vi "Set simulated or real mode.vi"(8 "error in (no error)":errorcluster, 11 "Channel in":refnum<class "SPARC4_Channel.lvclass">) -> (0 "error out":errorcluster, 3 "Channel out":refnum<class "SPARC4_Channel.lvclass">)   [LabVIEW 2018, in "SPARC4_Channel.lvclass"]
doc: "Choose between the simulated or real camera class"
uses:
  SPARC4_Channel.lvclass
  C:/Users/Denis/Desktop/S4ACS/S4ACS/Channel/Channel.lvclass
  Sim_Ixon_Ultra/Sim_Ixon_Ultra.lvclass
  C:/Users/Denis/Desktop/S4ACS/S4ACS/Sim_CCD/Sim_CCD.lvclass
  Ixon_Ultra/Ixon_Ultra.lvclass
  C:/Users/Denis/Desktop/S4ACS/S4ACS/Sim_Ixon_Ultra/Sim_Ixon_Ultra.lvclass
  Channel/Channel.lvclass
  Sim_CCD/Sim_CCD.lvclass
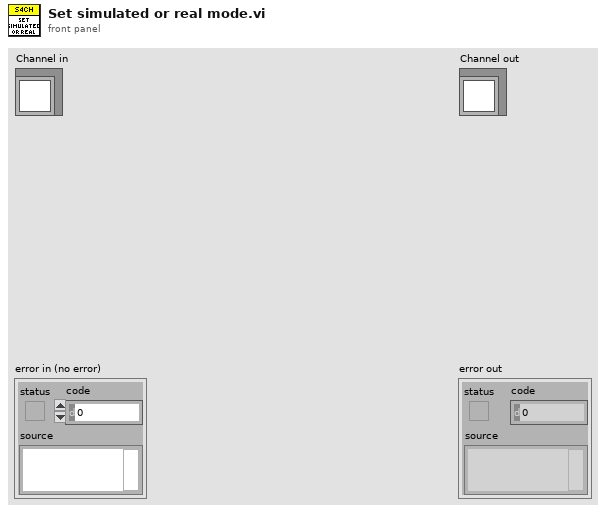
[diagram p1: front panel]
types:
  T1 = cluster{"Image path":path, "Channel":u8, "ACS mode":u16, "Log file path":path, "log level":u16}
  T2 = cluster{"State Machine.lvclass":refnum<class "State Machine.lvclass">, "RxTx.lvclass":refnum<class "RxTx.lvclass">, "Save_Header_RxTx.lvclass":refnum<class "RxTx.lvclass">, "Status SM.lvclass":refnum<class "State Machine.lvclass">, "Status RxTx.lvclass":refnum<class "RxTx.lvclass">, "servers array":refnum<class "Server.lvclass">[], "Events log file.lvclass":refnum<class "Log File.lvclass">, "Errors log file.lvclass":refnum<class "Log File.lvclass">, "Keywords log file.lvclass":refnum<class "Log File.lvclass">, "Sim_CCD.lvclass":refnum<class "Sim_CCD.lvclass">}
  T3 = cluster{"FRAMES_DONE":u16, "CCD_STATUS":string, "CURRENT_TEMPERATURE":i16, "TEMPERATURE_STATUS":string, "FRAME_EXPOSURE_TIME":dbl, "SERIAL_NUMBER":u16, "ACQUIRING":bool, "POWER":bool, "ACS MODE":bool}
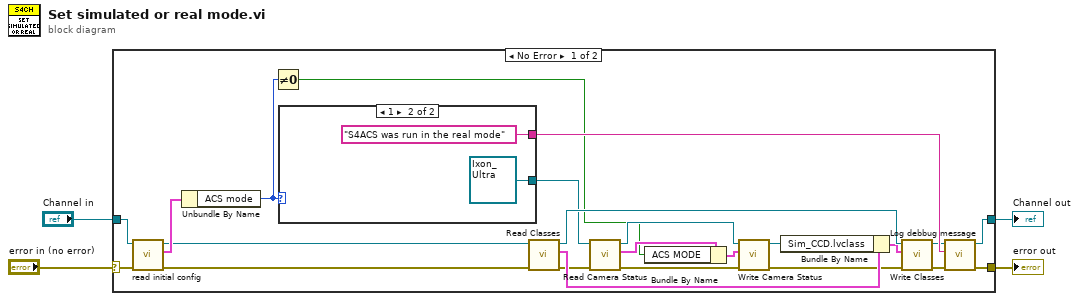
[diagram p0: block diagram]
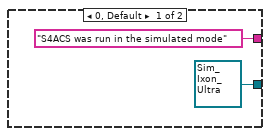
[diagram p2: hidden frame]
diagram:
  n1 = case shown="No Error" "error in (no error)" {
    selector: "error in (no error)" -> [w24 w33]
    tunnel: [w26 w33] -> w2
    tunnel: [w27 w32] -> w1
    tunnel: "Channel in" -> [w23 w32]
    frame No Error {
      n2 = call-dynamic "read initial config.vi"("error in (no error)"=w24, "Channel in"=w23) -> ("error out"=w20:errorcluster, "Configuration to initialize ACS"=w22:T1, "Channel out"=w21:refnum<class "SPARC4_Channel.lvclass">)  [unwired: 7 in]
      n3 = Unbundle By Name(w22) -> ("ACS mode"=w6:u16)
      n4 = Not Equal To 0?(x=w6) -> (x != 0?=w5:bool)
      n5 = case shown="1" w6 {
        tunnel: ["S4ACS was run in the simulated mode" ("String") "S4ACS was run in the real mode" ("String")] -> w25
        tunnel: [refnum<class "Sim_Ixon_Ultra.lvclass"> refnum ("Sim_Ixon_Ultra.lvclass") refnum<class "Ixon_Ultra.lvclass"> refnum ("Ixon_Ultra.lvclass")] -> w9
        frame 0, Default {
        }
        frame 1 {
        }
      }
      n6 = call-dynamic "Read Classes.vi"("error in (no error)"=w20, "Channel in"=w21) -> ("error out"=w14:errorcluster, "Classes"=w16:T2, "Channel out"=w19:refnum<class "SPARC4_Channel.lvclass">)  [unwired: 7 in]
      n7 = call "Read Camera Status.vi"("error in (no error)"=w14, "CCDCamera in"=w9) -> ("error out"=w13:errorcluster, "camera status"=w8:T3, "CCDCamera out"=w10:refnum<class "Sim_Ixon_Ultra.lvclass">)  [unwired: 7 in]
      n8 = Bundle By Name(cluster=w8, "ACS MODE"=w5) -> (w7:T3)
      n9 = call "Write Camera Status.vi"("error in (no error)"=w13, "camera status"=w7, "CCDCamera in"=w10) -> ("error out"=w12:errorcluster, "CCDCamera out"=w11:refnum<class "Sim_Ixon_Ultra.lvclass">)  [unwired: 7 in]
      n10 = Bundle By Name(cluster=w16, "Sim_CCD.lvclass"=w11) -> (w15:T2)
      n11 = call-dynamic "Write Classes.vi"("error in (no error)"=w12, "Classes"=w15, "Channel in"=w19) -> ("error out"=w17:errorcluster, "Channel out"=w18:refnum<class "SPARC4_Channel.lvclass">)  [unwired: 7 in]
      n12 = call "Log debbug message.vi"("error in (no error)"=w17, "String"=w25, "Channel in"=w18) -> ("error out"=w26:errorcluster, "Channel out"=w27:refnum<class "SPARC4_Channel.lvclass">)  [unwired: 7 in]
    }
    frame Error {
    }
  }
  "error out" <- w2
  "Channel out" <- w1
